vi "parseDataMote.vi"(3 "input data":string) -> (0 "source type (1 byte)":u8, 1 "node id (1 byte)":u8, 4 "Timestamp (19 bytes)":string, 5 "location":string, 6 "data 1 (2 bytes)":u16, 7 "data 2 (2 bytes)":u16, 8 "data 3 (2 bytes)":u16, 9 "data 4 (2 bytes)":u16)   [LabVIEW 2011]
panel:
  out "input data size (in bytes)":i32
  out "input data (in hex)":string[](array[string])
  # "Year"
  # "Month"
  # "Day"
  # "Hour"
  # "Min"
  # "Sec"
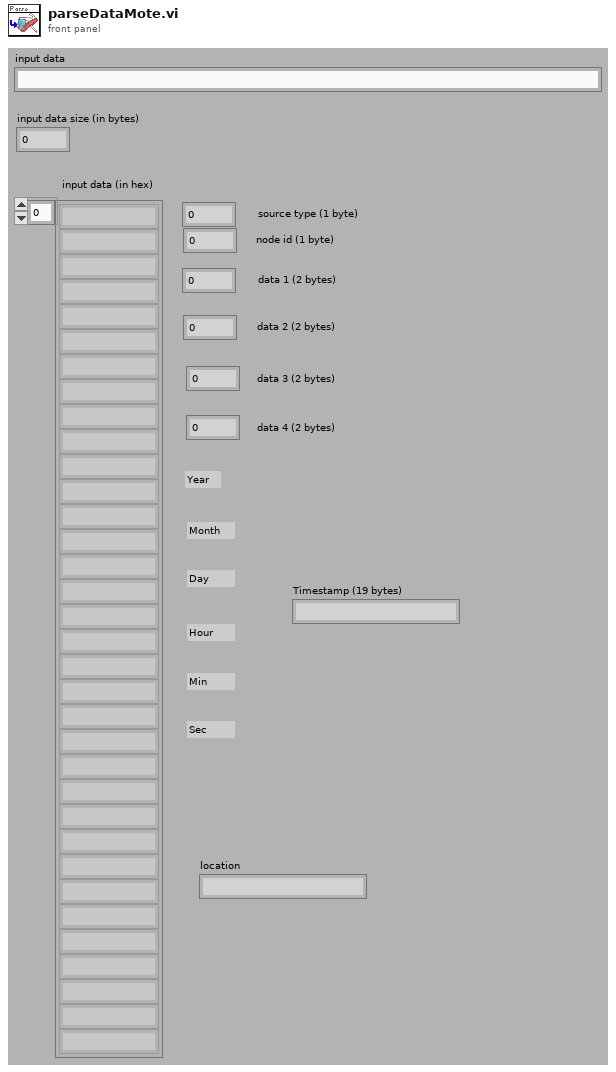
[diagram p1: front panel]
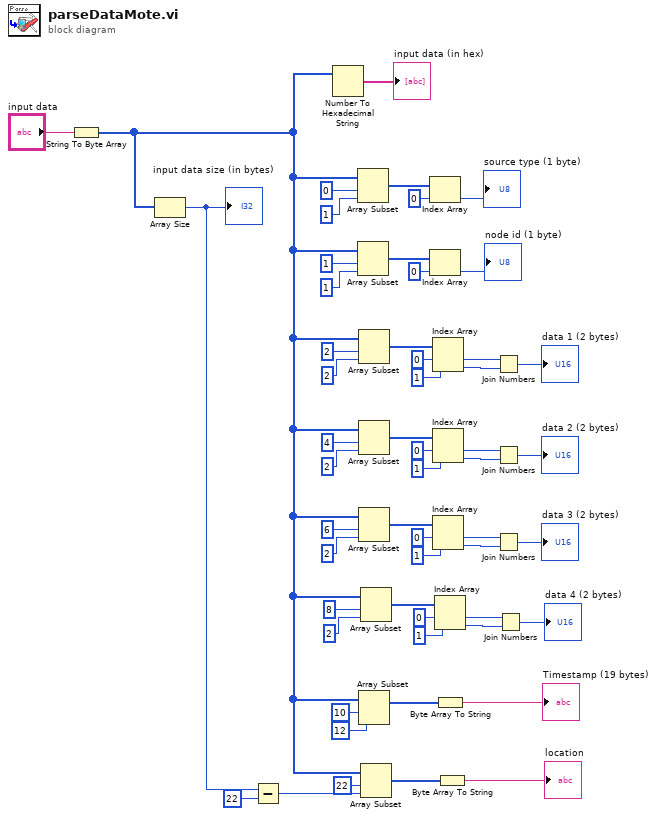
[diagram p0: block diagram]
diagram:
  n1 = String To Byte Array(string="input data") -> (unsigned byte array=w2:u8[])
  n2 = Array Size(array=w2) -> (size(s)=w12:i32)
  "input data size (in bytes)" <- w12
  n3 = Subtract(x=w12, y=22) -> (x-y=w10:i32)
  n4 = Number To Hexadecimal String(2:w2) -> (0:→"input data (in hex)":string[])  [unwired: 1 in]
  n5 = Array Subset(array=w2, index=0 ("x"), length=1 ("x")) -> (w48:u8[])
  n6 = Array Subset(array=w2, index=1 ("x"), length=1 ("x")) -> (w42:u8[])
  n7 = Array Subset(array=w2, index=2 ("x"), length=2 ("x")) -> (w45:u8[])
  n8 = Array Subset(array=w2, index=4 ("x"), length=2 ("x")) -> (w34:u8[])
  n9 = Array Subset(array=w2, index=6 ("x"), length=2 ("x")) -> (w26:u8[])
  n10 = Array Subset(array=w2, index=10, length=12) -> (w17:u8[])
  n11 = Array Subset(array=w2, index=8 ("x"), length=2 ("x")) -> (w5:u8[])
  n12 = Array Subset(array=w2, index=22, length=w10) -> (w13:u8[])
  n13 = Index Array(array=w48, index=0) -> (element=→"source type (1 byte)":u8)
  n14 = Index Array(array=w42, index=0) -> (element=→"node id (1 byte)":u8)
  n15 = Index Array(array=w45, index #1=0 ("index"), index #2=1 ("index")) -> (element #1=w39:u8, element #2=w38:u8)
  n16 = Index Array(array=w34, index #1=0 ("index"), index #2=1 ("index")) -> (element #1=w31:u8, element #2=w30:u8)
  n17 = Index Array(array=w26, index #1=0 ("index"), index #2=1 ("index")) -> (element #1=w23:u8, element #2=w22:u8)
  n18 = Index Array(array=w5, index #1=0 ("index"), index #2=1 ("index")) -> (element #1=w8:u8, element #2=w9:u8)
  n19 = Byte Array To String(unsigned byte array=w17) -> (string=→"Timestamp (19 bytes)":string)
  n20 = Byte Array To String(unsigned byte array=w13) -> (string=→"location":string)
  n21 = Join Numbers(hi=w39, lo=w38) -> ((hi.lo)=→"data 1 (2 bytes)":u16)
  n22 = Join Numbers(hi=w31, lo=w30) -> ((hi.lo)=→"data 2 (2 bytes)":u16)
  n23 = Join Numbers(hi=w23, lo=w22) -> ((hi.lo)=→"data 3 (2 bytes)":u16)
  n24 = Join Numbers(hi=w8, lo=w9) -> ((hi.lo)=→"data 4 (2 bytes)":u16)
